vi "FFT Sine test.vi"() -> ()   [LabVIEW 2013]
uses:
  <vilib>/Analysis/2dsp.llb/Real FFT.vi
  <vilib>/Analysis/NI_AALBase.lvlib
  <vilib>/Analysis/NI_AALPro.lvlib
panel:
  out "Waveform Graph 2":dbl[](graph)
  out "Waveform Graph":dbl[](graph)
  in  "tones":T1(array[cluster])=[{"frequency"=10.0, "amplitude"=1.0, "phase"=0.0}, {"frequency"=20.0, "amplitude"=0.1, "phase"=0.0}] {"phase" format="%0.2f"; "amplitude" format="%0.2p"; "frequency" format="%0.2p"}
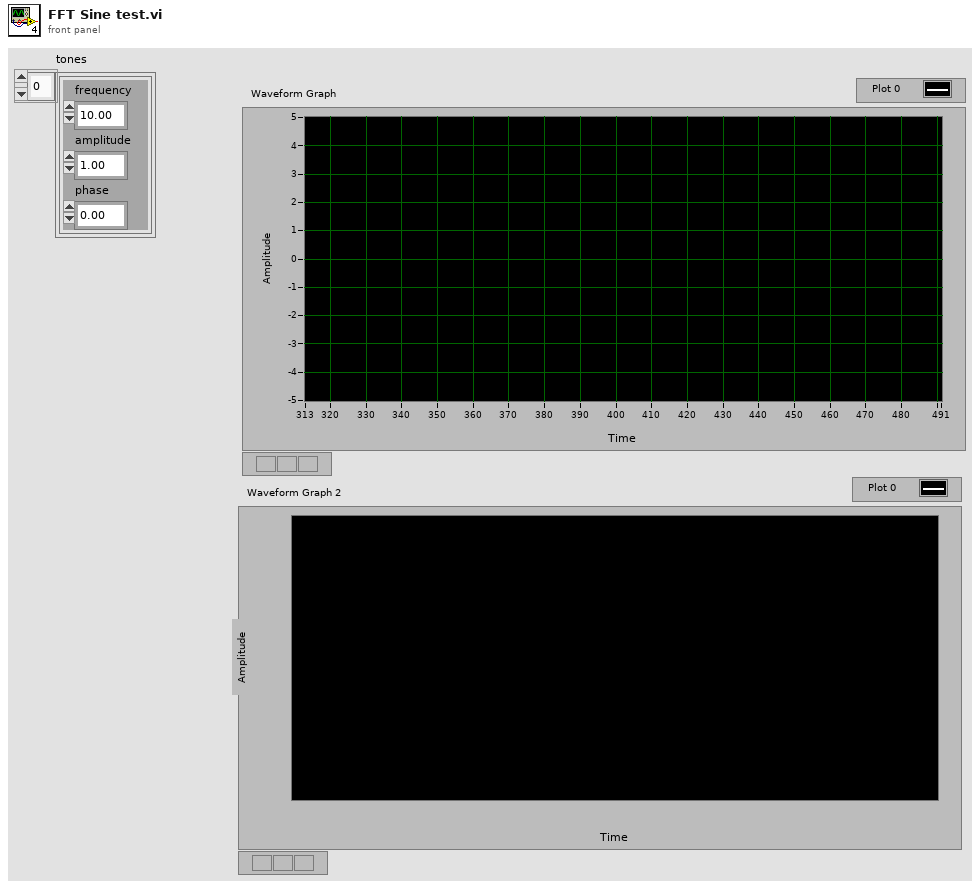
[diagram p1: front panel]
types:
  T1 = cluster{"frequency":dbl, "amplitude":dbl, "phase":dbl}[]
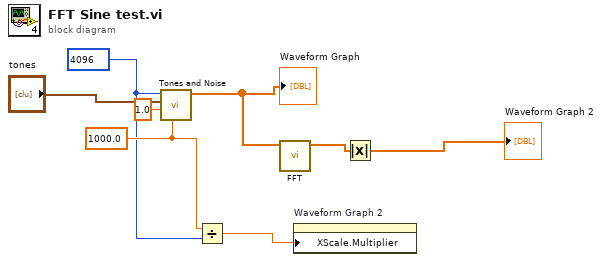
[diagram p0: block diagram]
diagram:
  w6 = 1000.0 ("Fs")
  w2 = 4096 ("samples")
  n1 = call <vilib>:"Tones and Noise.vi"("Fs"=w6, "noise (rms)"=1.0, "tones"="tones", "samples"=w2) -> ("tones and noise"=w7:dbl[])  [unwired: 6 in, 1 out]
  "Waveform Graph" <- w7
  n2 = Divide(x=w6, y=w2) -> (x/y=w5:dbl)
  n3 = call-poly <vilib>:"FFT.vi"("X"=w7) -> ("FFT {X}"=w4:cdb[])  [unwired: 9 in, 1 out]
  n4 = property on="Waveform Graph 2" class="WFGraph (strict)"("XScale.Multiplier"=w5) -> ()  [unwired: 2 in, 2 out]
  n5 = Absolute Value(x=w4) -> (abs(x)=→"Waveform Graph 2":dbl[])
